vi "rPi.vi"() -> ()   [LabVIEW 2020]
uses:
  <vilib>/Instr/_visa.llb/VISA Configure Serial Port (Instr).vi
  Subs/JSON_Formats.vi
panel:
  out "Cover":bool
  out "name":string
  in  "Write text":string
  in  "REPL":string
  in  "Connect":bool
  in  "Stop Button":bool
  in  "Port":refnum<visa-resource-name>
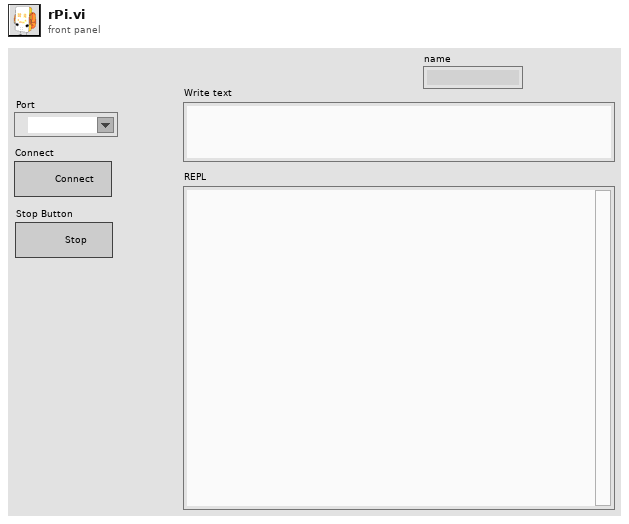
[diagram p1: front panel]
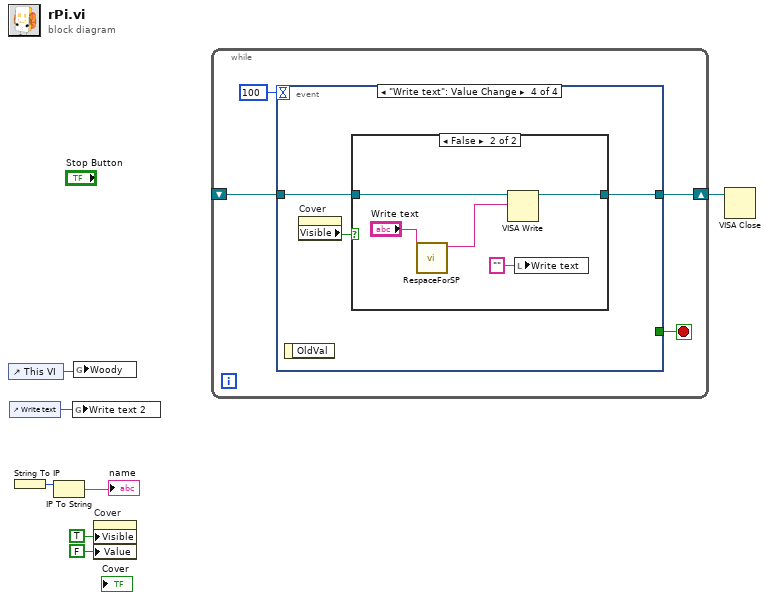
[diagram p0: block diagram]
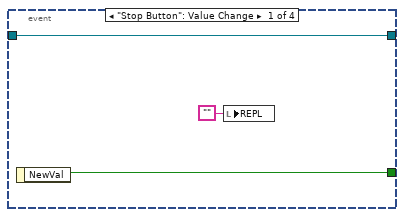
[diagram p2: hidden frame]
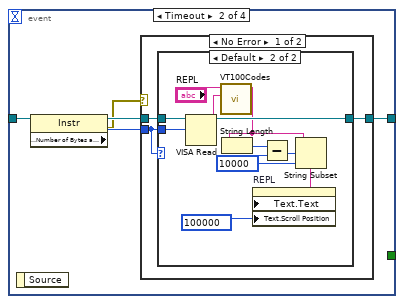
[diagram p3: hidden frame]
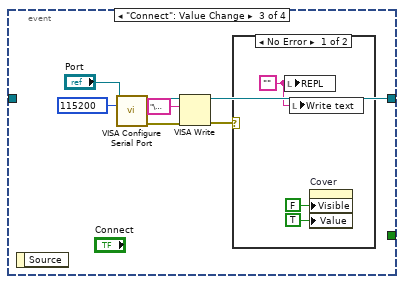
[diagram p6: hidden frame]
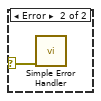
[diagram p7: hidden frame]
diagram:
  n1 = control-ref of="This VI"() -> (w2:refnum<vi>)
  n2 = control-ref of="Write text"() -> (w1:refnum<vi>)
  n3 = String To IP() -> (0:w7:u32)  [unwired: 1 in]
  n4 = IP To String(2:w7) -> (0:→"name":string)  [unwired: 1 in]
  n5 = global write "JSON_Formats.vi" "Write text 2"(w1) -> ()
  n6 = global write "JSON_Formats.vi" "Woody"(w2) -> ()
  n7 = property on="Cover" class="Bool (strict)"("Visible"=TRUE, "Value"=FALSE ("Cover")) -> ()  [unwired: 2 in, 2 out]
  n8 = while {
    shift-right: [w10] -> w3
    shift-left: _ -> [w9]
    stop <- w11 stop-if-true
    n9 = event shown="[3] \"Write text\": Value Change" {
      selector: _ -> [_ _ _ _]
      dyn-events: _ -> [_ _ _ _]
      timeout: 100 -> [_ _ _ _]
      tunnel: [w12 _ _ _] -> w11
      tunnel: [w13 w17 w38 w47] -> w10
      tunnel: w9 -> [w13 w16 _ w48]
      event "Stop Button": Value Change {
        n10 = event-data() -> ("NewVal"=w12:bool)  [unwired: 1 in]
        n11 = local write "REPL"("") -> ()
      }
      event Timeout {
        n12 = event-data() -> ()  [unwired: 1 in, 1 out]
        n13 = property class="Instr"(reference=w16) -> (error out=w15:errorcluster, "Serial Settings:Number of Bytes at Serial Port"=w18:u32)  [unwired: 1 in, 1 out]
        n14 = case shown="No Error" w15 {
          tunnel: w18 -> [w19 _]
          tunnel: [w21 w34] -> w17
          tunnel: w16 -> [w20 w34]
          frame No Error {
            n15 = case shown="Default" w19 {
              tunnel: w19 -> [_ w33]
              tunnel: [w22 w32] -> w21
              tunnel: w20 -> [w22 w31]
              frame 0 {
              }
              frame Default {
                w25 = 10000 ("length (rest)")
                n16 = VISA Read(VISA resource name=w31, byte count=w33) -> (VISA resource name out=w32:refnum<visa-resource-name>, read buffer=w27:string)  [unwired: 1 in, 2 out]
                n17 = call "VT100Codes.vi"("read buffer"=w27, "Console In"="REPL") -> ("Console Out"=w23:string)  [unwired: 9 in]
                n18 = String Length(string=w23) -> (length=w26:i32)
                n19 = Subtract(x=w26, y=w25) -> (x-y=w24:i32)
                n20 = String Subset(string=w23, offset (0)=w24, length (rest)=w25) -> (substring=w29:string)
                n21 = property on="REPL" class="Str"("Text.Text"=w29, "Text.Scroll Position"=u32 100000 ("Text.Selection:Start")) -> ()  [unwired: 2 in, 2 out]
              }
            }
          }
          frame Error {
          }
        }
      }
      event "Connect": Value Change {
        n22 = event-data() -> ()  [unwired: 1 in, 1 out]
        n23 = call-poly "VISA Configure Serial Port"("VISA resource name"="Port", "baud rate (9600)"=u32 115200) -> ("VISA resource name out"=w39:refnum<visa-resource-name>, "error out"=w36:errorcluster)  [unwired: 12 in]
        n24 = VISA Write(VISA resource name=w39, write buffer="\u0003", error in (no error)=w36) -> (VISA resource name out=w38:refnum<visa-resource-name>, error out=w35:errorcluster)  [unwired: 1 out]
        n25 = case shown="No Error" w35 {
          selector: w35 -> [_ w45]
          frame No Error {
            w44 = ""
            n26 = local write "REPL"(w44) -> ()
            n27 = local write "Write text"(w44) -> ()
            n28 = property on="Cover" class="Bool (strict)"("Visible"=FALSE, "Value"=TRUE ("Cover")) -> ()  [unwired: 2 in, 2 out]
          }
          frame Error {
            n29 = call <vilib>:"Simple Error Handler.vi"("error in (no error)"=w45) -> ()  [unwired: 4 in, 5 out]
          }
        }
      }
      event "Write text": Value Change {
        n30 = event-data() -> ()  [unwired: 1 in, 1 out]
        n31 = property on="Cover" class="Bool (strict)"() -> ("Visible"=w46:bool)  [unwired: 2 in, 2 out]
        n32 = case shown="False" w46 {
          tunnel: w48 -> [w49 w54]
          tunnel: [w49 w53] -> w47
          frame True {
          }
          frame False {
            n33 = call "RespaceForSP.vi"("Code"="Write text") -> ("Cleaned for SPIKE"=w50:string)  [unwired: 10 in]
            n34 = VISA Write(VISA resource name=w54, write buffer=w50) -> (VISA resource name out=w53:refnum<visa-resource-name>)  [unwired: 1 in, 2 out]
            n35 = local write "Write text"("" ("Write text")) -> ()
          }
        }
      }
    }
  }
  n36 = VISA Close(VISA resource name=w3) -> ()  [unwired: 1 in, 1 out]
